vi "Draw Line v2.vi"(6 "Colour":u32(colorbox), 9 "Point 2":T1, 10 "Point 1":T1, 11 "Pixel Data in":u32[][](array[numeric])) -> (3 "Pixel Data out":u32[][](array[numeric]))   [LabVIEW 2022 SP3, in "Raster.lvlib"]
uses:
  Raster.lvlib
  Point 2D (I32).ctl
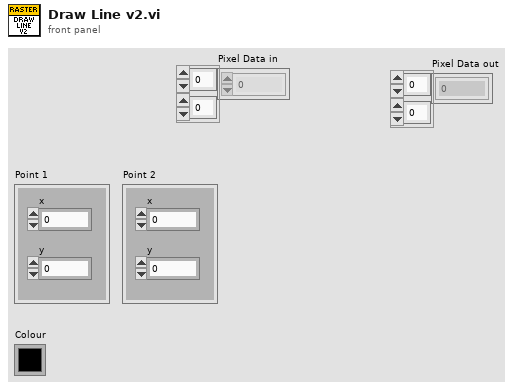
[diagram p1: front panel]
types:
  T1 = typedef "Raster.lvlib/Point 2D (I32).ctl" = cluster{"x":i32, "y":i32}
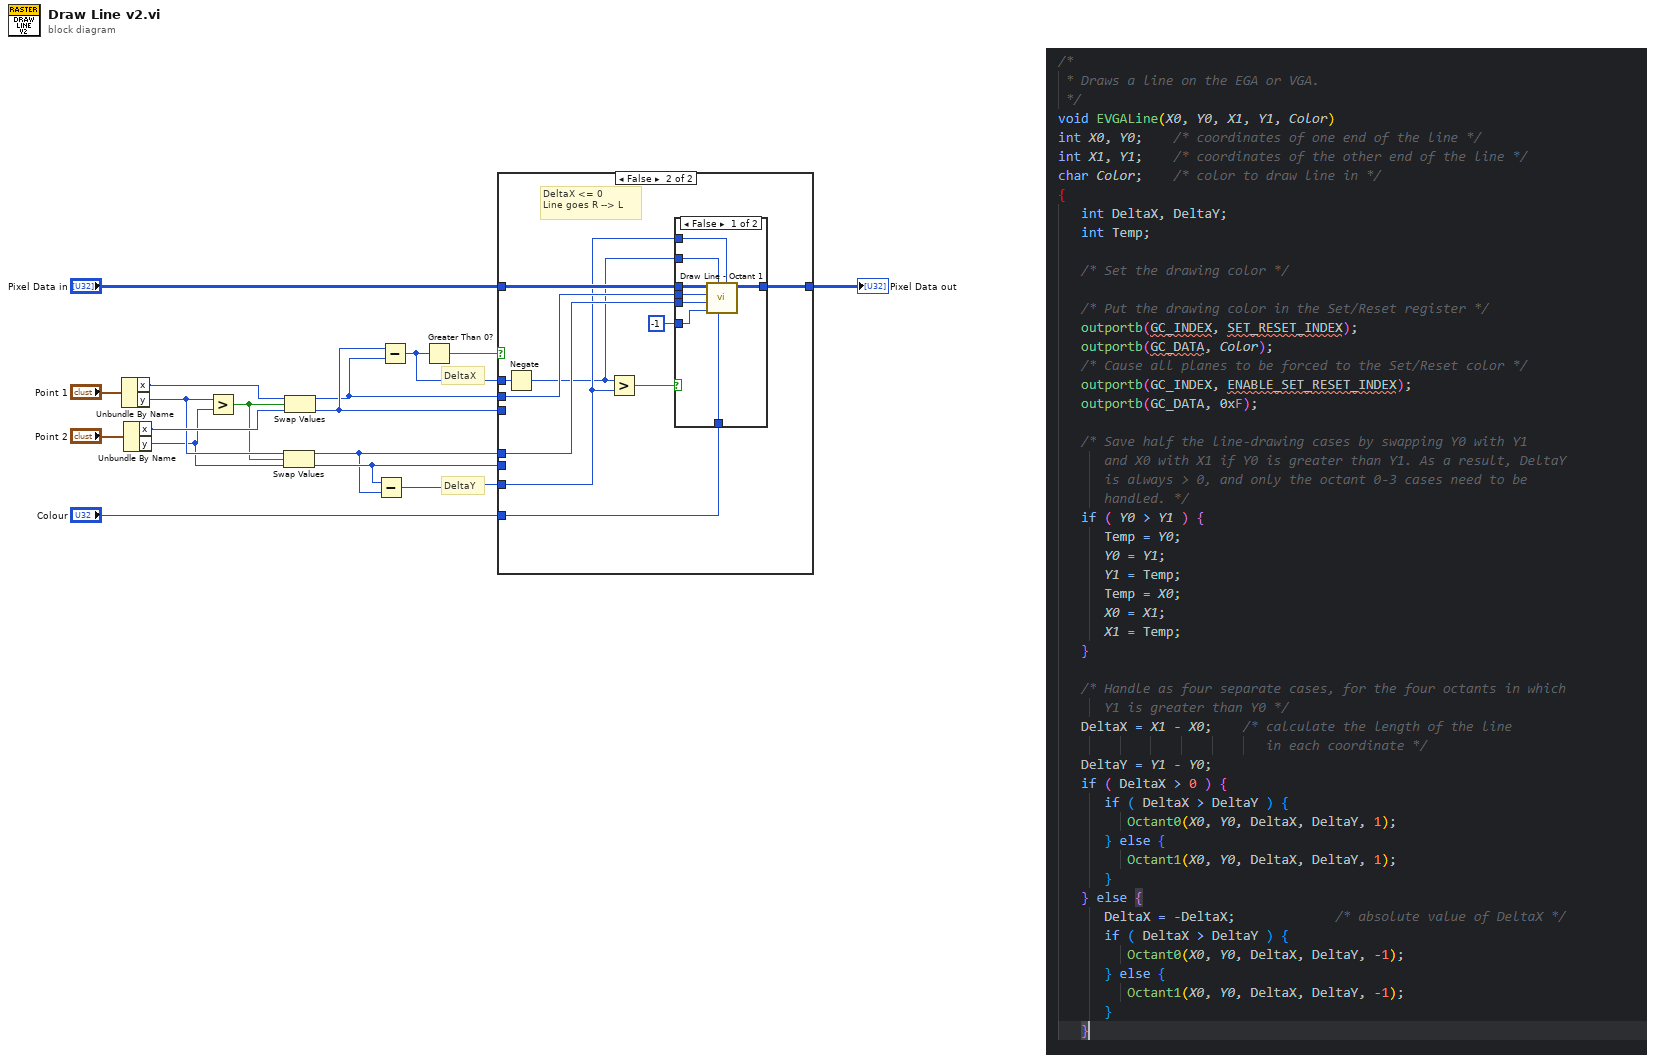
[diagram p0: block diagram]
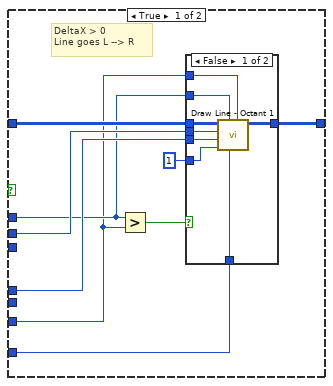
[diagram p2: hidden frame]
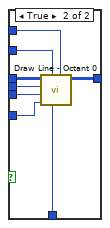
[diagram p3: hidden frame]
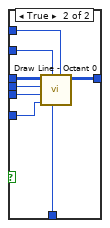
[diagram p4: hidden frame]
diagram:
  # "DeltaY"
  # "DeltaX"
  n1 = Unbundle By Name("Point 1") -> ("x"=w14:i32, "y"=w12:i32)
  n2 = Unbundle By Name("Point 2") -> ("x"=w13:i32, "y"=w10:i32)
  n3 = Greater?(x=w12, y=w10) -> (0:w11:bool)
  n4 = Swap Values(12:w12, 13:w11, 14:w10) -> (1:w6:i32, 3:w7:i32)
  n5 = Swap Values(12:w14, 13:w11, 14:w13) -> (1:w8:i32, 3:w9:i32)
  n6 = Subtract(x=w7, y=w6) -> (x-y=w4:i32)
  n7 = Subtract(x=w9, y=w8) -> (x-y=w3:i32)
  n8 = Greater Than 0?(x=w3) -> (x > 0?=w5:bool)
  n9 = case shown="False" w5 {
    tunnel: "Pixel Data in" -> [w26 w52]
    tunnel: [w25 w51] -> w2
    tunnel: "Colour" -> [w24 w50]
    tunnel: w8 -> [w23 w49]
    tunnel: w9 -> [_ _]
    tunnel: w6 -> [w22 w48]
    tunnel: w7 -> [_ _]
    tunnel: w4 -> [w18 w44]
    tunnel: w3 -> [w19 w45]
    frame True {
      # "DeltaX > 0\nLine goes L --> R"
      n10 = Greater?(x=w19, y=w18) -> (0:w21:bool)
      n11 = case shown="False" w21 {
        tunnel: w26 -> [w34 w42]
        tunnel: [w33 w41] -> w25
        tunnel: w24 -> [w32 w35]
        tunnel: w23 -> [w31 w39]
        tunnel: w22 -> [w30 w38]
        tunnel: 1 ("x Direction") -> [w29 w40]
        tunnel: w19 -> [w28 w37]
        tunnel: w18 -> [w27 w36]
        frame False {
          n12 = call "Draw Line - Octant 1.vi"("Delta y"=w27, "Colour"=w32, "Delta x"=w28, "x Direction"=w29, "Y0"=w30, "X0"=w31, "Pixel Data in"=w34) -> ("Pixel Data out"=w33:u32[][])  [unwired: 4 in]
        }
        frame True {
          n13 = call "Draw Line - Octant 0.vi"("Delta y"=w36, "Colour"=w35, "Delta x"=w37, "x Direction"=w40, "Y0"=w38, "X0"=w39, "Pixel Data in"=w42) -> ("Pixel Data out"=w41:u32[][])  [unwired: 4 in]
        }
      }
    }
    frame False {
      # "DeltaX <= 0\nLine goes R --> L"
      n14 = Negate(x=w45) -> (-x=w43:i32)
      n15 = Greater?(x=w43, y=w44) -> (0:w47:bool)
      n16 = case shown="False" w47 {
        tunnel: w52 -> [w60 w68]
        tunnel: [w59 w67] -> w51
        tunnel: w50 -> [w58 w61]
        tunnel: w49 -> [w57 w65]
        tunnel: w48 -> [w56 w64]
        tunnel: -1 ("x Direction") -> [w55 w66]
        tunnel: w43 -> [w54 w63]
        tunnel: w44 -> [w53 w62]
        frame False {
          n17 = call "Draw Line - Octant 1.vi"("Delta y"=w53, "Colour"=w58, "Delta x"=w54, "x Direction"=w55, "Y0"=w56, "X0"=w57, "Pixel Data in"=w60) -> ("Pixel Data out"=w59:u32[][])  [unwired: 4 in]
        }
        frame True {
          n18 = call "Draw Line - Octant 0.vi"("Delta y"=w62, "Colour"=w61, "Delta x"=w63, "x Direction"=w66, "Y0"=w64, "X0"=w65, "Pixel Data in"=w68) -> ("Pixel Data out"=w67:u32[][])  [unwired: 4 in]
        }
      }
    }
  }
  "Pixel Data out" <- w2
